vi "RTHost.vi"() -> ()   [LabVIEW 2013]
uses:
  <vilib>/Platform/TimedLoop/XDataNode/timing_clust.ctl
  <vilib>/Platform/TimedLoop/XDataNode/nitl_modes.ctl
  <vilib>/Platform/TimedLoop/XDataNode/wakeup.ctl
  <vilib>/FPGAPlugInAG/sbRIO-9632/niLvFpga_Open_sbRIO-9632.vi
  <vilib>/Utility/error.llb/Error Cluster From Error Code.vi
  <vilib>/rvi/errors/niLvFpgaAdjustHostInterfaceError.vi
  <vilib>/FPGAPlugInAG/sbRIO-9632/niLvFpga_Close_sbRIO-9632.vi
  <vilib>/rvi/interface/nirviOpenFPGA/nirviOpenFPGA.xnode
  FPGA Bitfiles/VMS15_FPGATarget_RTHost_xaXps4HcxjY.lvbitx
  <vilib>/rvi/interface/nirviReadWriteControl/nirviReadWriteControl.xnode
  <vilib>/Platform/TimedLoop/XDataNode/XDataNode.xnode
  <vilib>/rvi/interface/nirviCloseFPGA/nirviCloseFPGA.xnode
  NiFpgaLv.dll
  <vilib>/Platform/TimedLoop/XDataNode/XDNodeRunTimeDep.lvlib
panel:
  out "电池过温":bool
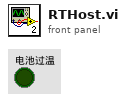
[diagram p1: front panel]
types:
  T1 = typedef "XDNodeRunTimeDep.lvlib/timing_clust.ctl" = cluster{"Expected End [f-1]":u64, "Actual End [f-1]":u64, "Finished Late? [f-1]":bool, "Expected End [i-1]":u64, "Actual End [i-1]":u64, "Finished Late? [i-1]":bool, "Expected Start [i]":u64, "Actual Start [i]":u64, "Expected Start [f]":u64, "Actual Start [f]":u64, "Source Name":string, "Structure Name":string, "Period":i64, "Deadline":i64, "Offset":i64, "Start":i64, "Priority":i32, "Timeout":i32, "Mode":T2, "Wakeup Reason":T3, "Error":errorcluster, "Source Type":string, "Secondary Source Type":string, "Global End Time":u64, "Global Start Time":u64, "Frame Duration":u64, "Iteration Duration":u64, "Assigned CPU":i32, "I/O Scan Engine Mode":u32}
  T2 = typedef "XDNodeRunTimeDep.lvlib/nitl_modes.ctl" = enum32{"No Change", "Process missed periods, maintain original phase", "Discard missed periods, maintain original phase", "Process missed periods, ignore original phase", "Discard missed periods, ignore original phase"}
  T3 = typedef "XDNodeRunTimeDep.lvlib/wakeup.ctl" = enum32{"Normal", "Aborted", "Asynchronous wakeup", "Timing source error", "Timed loop error", "Timeout"}
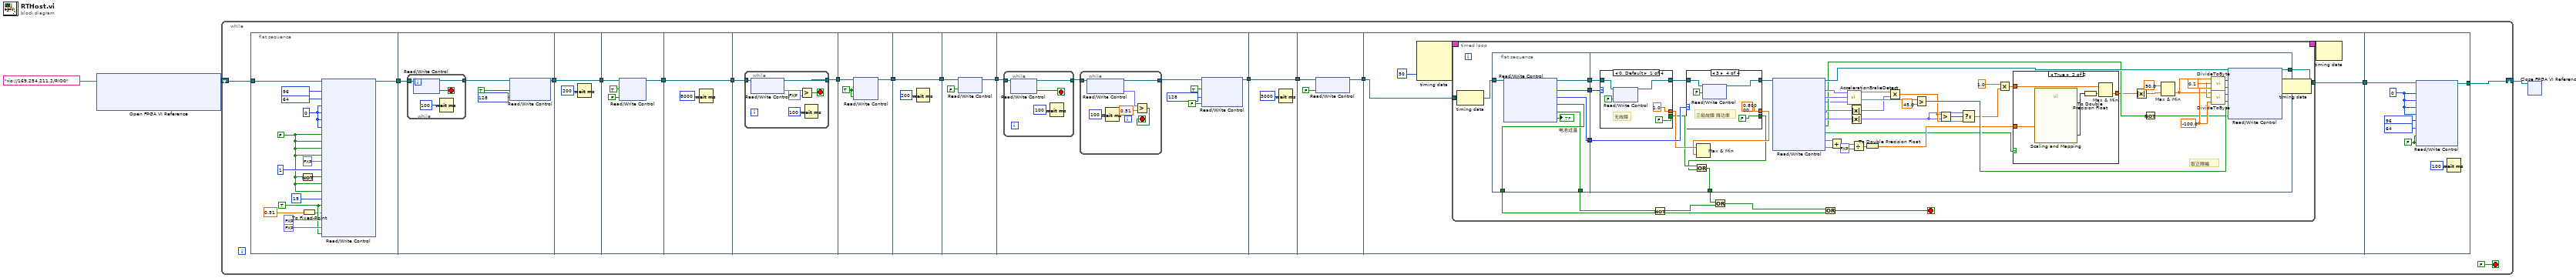
[diagram p0: block diagram]
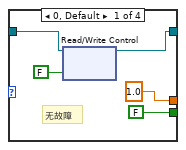
[diagram p3: hidden frame]
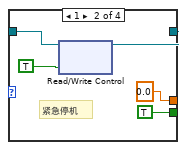
[diagram p4: hidden frame]
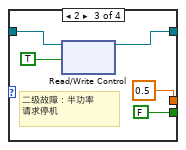
[diagram p5: hidden frame]
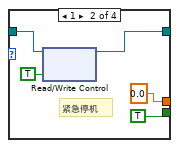
[diagram p6: hidden frame]
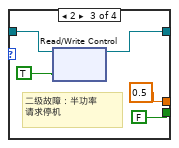
[diagram p7: hidden frame]
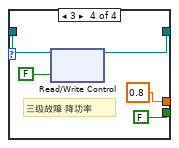
[diagram p8: hidden frame]
diagram:
  n1 = xnode "Open FPGA VI Reference"("resource name"=tag "rio://169.254.211.2/RIO0") -> ("FPGA VI Reference Out"=w1:refnum<k20>)  [unwired: 1 in, 1 out]
  n2 = while {
    shift-right: [w4] -> w2
    shift-left: w1 -> [w19]
    stop <- FALSE stop-if-true
    n3 = flat-sequence {
      tunnel: w19 -> [w31]
      tunnel: [w30] -> w18
      tunnel: w18 -> [w36]
      tunnel: [w35] -> w17
      tunnel: w17 -> [w45]
      tunnel: [w45] -> w16
      tunnel: w16 -> [w48]
      tunnel: [w47] -> w15
      tunnel: w15 -> [w51]
      tunnel: [w51] -> w10
      tunnel: [w53] -> w14
      tunnel: w10 -> [w52]
      tunnel: w14 -> [w62]
      tunnel: [w61] -> w7
      tunnel: w7 -> [w64]
      tunnel: [w64] -> w6
      tunnel: w6 -> [w67]
      tunnel: [w66] -> w5
      tunnel: w5 -> [w74]
      tunnel: [w69] -> w13
      tunnel: w13 -> [w86]
      tunnel: [w86] -> w9
      tunnel: [w88] -> w12
      tunnel: w9 -> [w89]
      tunnel: w12 -> [w92]
      tunnel: [w91] -> w11
      tunnel: w11 -> [w217]
      tunnel: [w212] -> w4
      frame #0 {
        w24 = TRUE ("AMS")
        w33 = u8 0 ("Byte 7")
        w23 = FALSE ("MotorAlarm?")
        n4 = Not(x=w23) -> (.not. x?=w22:bool)
        n5 = To Fixed-Point(number=0.51) -> (fixed-point=w21:fxp<+/-,32,16>)  [unwired: 1 in]
        n6 = xnode "Read/Write Control"("FPGA VI Reference In"=w31, "MCCmdByte"=u8 96, "BMCmdByte"=u8 64, "MC1TqSet_L"=w33, "MC1TqSet_H"=w33, "MC2TqSet_L"=w33, "MC2TqSet_H"=w33, "PREO"=w23, "AIRPO"=w23, "AIRNO"=w23, "BRAKELO"=w23, "开风扇温度值"=fxp<+,8,6> 40.0, "发送间隔(mSec)"=u8 1, "AMS"=w22, "BA"=w23, "MA"=w23, "接收窗口(mSec)"=u8 19, "Ready"=w24, "刹车标定上限"=w21, "PowerPermitted"=fxp<+/-,64,32> 60.0, "开水泵温度值"=fxp<+/-,32,16> 60.0, "ErrorMonitoring?"=w24) -> ("FPGA VI Reference Out"=w30:refnum<k20>)  [unwired: 1 in, 1 out]
      }
      frame #1 {
        n7 = while {
          tunnel: w36 -> [w43]
          tunnel: [w42] -> w37
          stop <- w40 stop-if-true
          n8 = xnode "Read/Write Control"("FPGA VI Reference In"=w43) -> ("FPGA VI Reference Out"=w42:refnum<k20>, "Start？"=w40:bool)  [unwired: 1 in, 1 out]
          n9 = Wait (ms)(milliseconds to wait=u32 100) -> ()  [unwired: 1 out]
        }
        n10 = xnode "Read/Write Control"("FPGA VI Reference In"=w37, "PREO"=TRUE, "BMCmdByte"=u8 128) -> ("FPGA VI Reference Out"=w35:refnum<k20>)  [unwired: 1 in, 1 out]
      }
      frame #2 {
        n11 = Wait (ms)(milliseconds to wait=u32 200) -> ()  [unwired: 1 out]
      }
      frame #3 {
        n12 = xnode "Read/Write Control"("FPGA VI Reference In"=w48, "AIRNO"=TRUE, "Ready"=FALSE) -> ("FPGA VI Reference Out"=w47:refnum<k20>)  [unwired: 1 in, 1 out]
      }
      frame #4 {
        n13 = Wait (ms)(milliseconds to wait=u32 8000) -> ()  [unwired: 1 out]
      }
      frame #5 {
        n14 = while {
          tunnel: [w59] -> w53
          tunnel: w52 -> [w56]
          stop <- w54 stop-if-true
          n15 = xnode "Read/Write Control"("FPGA VI Reference In"=w56) -> ("FPGA VI Reference Out"=w59:refnum<k20>, "MC1VinIs"=w57:fxp<+/-,32,16>)  [unwired: 1 in, 1 out]
          n16 = Greater?(x=w57, y=fxp<+,18,10> 480.0) -> (0:w54:bool)
          n17 = Wait (ms)(milliseconds to wait=u32 100) -> ()  [unwired: 1 out]
        }
      }
      frame #6 {
        w60 = TRUE ("AIRPO")
        n18 = xnode "Read/Write Control"("FPGA VI Reference In"=w62, "AIRPO"=w60, "Ready"=w60) -> ("FPGA VI Reference Out"=w61:refnum<k20>)  [unwired: 1 in, 1 out]
      }
      frame #7 {
        n19 = Wait (ms)(milliseconds to wait=u32 200) -> ()  [unwired: 1 out]
      }
      frame #8 {
        n20 = xnode "Read/Write Control"("FPGA VI Reference In"=w67, "PREO"=FALSE) -> ("FPGA VI Reference Out"=w66:refnum<k20>)  [unwired: 1 in, 1 out]
      }
      frame #9 {
        n21 = while {
          tunnel: w74 -> [w78]
          tunnel: [w77] -> w73
          stop <- w75 stop-if-true
          n22 = xnode "Read/Write Control"("FPGA VI Reference In"=w78) -> ("FPGA VI Reference Out"=w77:refnum<k20>, "Start？"=w75:bool)  [unwired: 1 in, 1 out]
          n23 = Wait (ms)(milliseconds to wait=u16 100) -> ()  [unwired: 1 out]
        }
        n24 = while {
          tunnel: w73 -> [w82]
          tunnel: [w81] -> w72
          stop <- w79 stop-if-true
          n25 = xnode "Read/Write Control"("FPGA VI Reference In"=w82) -> ("FPGA VI Reference Out"=w81:refnum<k20>, "SIG_BRAKE"=w80:fxp<+/-,30,9>)  [unwired: 1 in, 1 out]
          n26 = Wait (ms)(milliseconds to wait=u16 100) -> ()  [unwired: 1 out]
          n27 = Greater?(x=w80, y=0.51) -> (0:w79:bool)
        }
        n28 = xnode "Read/Write Control"("FPGA VI Reference In"=w72, "BUZZERO"=TRUE, "MCCmdByte"=u8 128 ("CAN 4"), "Ready"=FALSE) -> ("FPGA VI Reference Out"=w69:refnum<k20>)  [unwired: 1 in, 1 out]
      }
      frame #10 {
        n29 = Wait (ms)(milliseconds to wait=u32 3000) -> ()  [unwired: 1 out]
      }
      frame #11 {
        n30 = xnode "Read/Write Control"("FPGA VI Reference In"=w89, "BUZZERO"=FALSE) -> ("FPGA VI Reference Out"=w88:refnum<k20>)  [unwired: 1 in, 1 out]
      }
      frame #12 {
        n31 = node-c288(i64 50 ("Period")) -> (w94:T1)  [unwired: 3 in]
        n32 = timed-loop {
          timing: w94 -> [_]
          timing-out: [_] -> w93
          tunnel: w92 -> [w104]
          tunnel: [w105] -> w91
          stop <- w96 stop-if-true
          n33 = node-c288() -> ()  [unwired: 1 in, 1 out]
          n34 = flat-sequence {
            tunnel: w104 -> [w109]
            tunnel: [w108] -> w100
            tunnel: [w112] -> w103
            tunnel: [w111] -> w102
            tunnel: [w110] -> w101
            tunnel: [w107] -> w98
            tunnel: w103 -> [w159]
            tunnel: w102 -> [w157]
            tunnel: w101 -> [w142]
            tunnel: [w143] -> w105
            tunnel: [w119] -> w99
            frame #0 {
              n35 = xnode "Read/Write Control"("FPGA VI Reference In"=w109) -> ("FPGA VI Reference Out"=w110:refnum<k20>, "BatteryErrorRank"=w112:u8, "MotorErrorRank"=w111:u8, "Stop？"=w108:bool, "SHTD"=w107:bool, "电池过温"=→"电池过温":bool)  [unwired: 1 in, 1 out]
            }
            frame #1 {
              w150 = -100.0 ("Offset")
              w149 = 0.1 ("Resolution")
              # "取正限幅"
              n36 = case shown="0, Default" w159 {
                tunnel: [1.0 0.0 sgl 0.5 0.8] -> w156
                tunnel: [FALSE TRUE FALSE FALSE] -> w154
                tunnel: [w188 w192 w196 w201] -> w158
                tunnel: w142 -> [w187 w193 w197 w202]
                frame 0, Default {
                  # "无故障"
                  n37 = xnode "Read/Write Control"("FPGA VI Reference In"=w187, "BA"=FALSE ("Alarm")) -> ("FPGA VI Reference Out"=w188:refnum<k20>)  [unwired: 1 in, 1 out]
                }
                frame 1 {
                  # "紧急停机"
                  n38 = xnode "Read/Write Control"("FPGA VI Reference In"=w193, "BA"=TRUE) -> ("FPGA VI Reference Out"=w192:refnum<k20>)  [unwired: 1 in, 1 out]
                }
                frame 2 {
                  # "二级故障：半功率\n请求停机"
                  n39 = xnode "Read/Write Control"("FPGA VI Reference In"=w197, "BA"=TRUE ("Alarm")) -> ("FPGA VI Reference Out"=w196:refnum<k20>)  [unwired: 1 in, 1 out]
                }
                frame 3 {
                  # "三级故障 降功率"
                  n40 = xnode "Read/Write Control"("FPGA VI Reference In"=w202, "BA"=FALSE ("Alarm")) -> ("FPGA VI Reference Out"=w201:refnum<k20>)  [unwired: 1 in, 1 out]
                }
              }
              n41 = case shown="3" w157 {
                tunnel: [1.0 0.0 sgl 0.5 sgl 0.8] -> w155
                tunnel: [w169 w175 w179 w183] -> w152
                tunnel: [FALSE TRUE FALSE FALSE] -> w153
                tunnel: w158 -> [w166 w173 w176 w181]
                frame 0, Default {
                  # "无故障"
                  n42 = xnode "Read/Write Control"("FPGA VI Reference In"=w166, "MA"=FALSE ("Alarm")) -> ("FPGA VI Reference Out"=w169:refnum<k20>)  [unwired: 1 in, 1 out]
                }
                frame 1 {
                  # "紧急停机"
                  n43 = xnode "Read/Write Control"("FPGA VI Reference In"=w173, "MA"=TRUE) -> ("FPGA VI Reference Out"=w175:refnum<k20>)  [unwired: 1 in, 1 out]
                }
                frame 2 {
                  # "二级故障：半功率\n请求停机"
                  n44 = xnode "Read/Write Control"("FPGA VI Reference In"=w176, "MA"=TRUE ("Alarm")) -> ("FPGA VI Reference Out"=w179:refnum<k20>)  [unwired: 1 in, 1 out]
                }
                frame 3 {
                  # "三级故障 降功率"
                  n45 = xnode "Read/Write Control"("FPGA VI Reference In"=w181, "MA"=FALSE ("Alarm")) -> ("FPGA VI Reference Out"=w183:refnum<k20>)  [unwired: 1 in, 1 out]
                }
              }
              n46 = Or(x=w154, y=w153) -> (x .or. y?=w119:bool)
              n47 = Max & Min(x=w156, y=w155) -> ()  [unwired: 2 out]
              n48 = xnode "Read/Write Control"("FPGA VI Reference In"=w152) -> ("FPGA VI Reference Out"=w141:refnum<k20>, "SIG_ACC1"=w138:fxp<+/-,30,9>, "SIG_ACC2"=w137:fxp<+/-,30,9>, "SIG_BRAKE"=w117:fxp<+/-,30,9>, "PowerLimited"=w139:fxp<+/-,16,6>, "TorquePermitted"=w133:fxp<+/-,64,40>, "SWT3?"=w131:bool, "SWT4?"=w128:bool, "MC2SpIs"=w127:fxp<+/-,32,16>, "MC1SpIs"=w126:fxp<+/-,32,16>)  [unwired: 1 in, 1 out]
              n49 = Add(x=w127, y=w126) -> (x+y=w125:fxp<+/-,33,17>)
              n50 = call "AccelerationBrakeDetect.vi"("油门1输入"=w138, "油门2输入"=w137, "刹车输入"=w117) -> ("油门1"=w140:dbl, "刹车"=w144:dbl)  [unwired: 3 out]
              n51 = Absolute Value(x=w139) -> (abs(x)=w115:fxp<+,16,6>)
              n52 = Absolute Value(x=w133) -> (abs(x)=w116:fxp<+,64,40>)
              n53 = Divide(x=w125, y=fxp<+/-,33,17> 2.0) -> (x/y=w123:fxp<+/-,64,34>)
              n54 = To Double Precision Float(number=w123) -> (double precision float=w130:dbl)
              n55 = Multiply(x=w140, y=w115) -> (x*y=w135:dbl)
              n56 = Greater?(x=w144, y=45.0) -> (0:w136:bool)
              n57 = Greater?(x=w135, y=w116) -> (0:w134:bool)
              n58 = Select(t=w116, s=w134, f=w135) -> (s? t:f=w132:dbl)
              n59 = Multiply(x=1.0, y=w132) -> (x*y=w129:dbl)
              n60 = case shown="True" w128 {
                tunnel: w130 -> [_ w165]
                tunnel: w129 -> [w160 w161]
                tunnel: [w160 w162] -> w122
                frame False {
                }
                frame True {
                  n61 = call "Scaling and Mapping"("Signals"=w165) -> ("Scaled Signals"=w163:dynamicdata)  [unwired: 9 in, 1 out]
                  n62 = To Double Precision Float(number=w163) -> (double precision float=w164:dbl)
                  n63 = Max & Min(x=w161, y=w164) -> (min(x,y)=w162:dbl)  [unwired: 1 out]
                }
              }
              n64 = Absolute Value(x=w122) -> (abs(x)=w120:dbl)
              n65 = Not(x=w131) -> (.not. x?=w118:bool)
              n66 = Max & Min(x=90.0, y=w120) -> (min(x,y)=w114:dbl)  [unwired: 1 out]
              n67 = call "DivideToByte.vi"("Offset"=w150, "Resolution"=w149, "Value"=w114) -> ("HighByte"=w145:u8, "LowByte"=w148:u8)
              n68 = call "DivideToByte.vi"("Offset"=w150, "Resolution"=w149, "Value"=w114) -> ("HighByte"=w146:u8, "LowByte"=w147:u8)
              n69 = xnode "Read/Write Control"("FPGA VI Reference In"=w141, "MC1TqSet_L"=w148, "MC1TqSet_H"=w145, "MC2TqSet_L"=w147, "MC2TqSet_H"=w146, "BRAKELO"=w136, "ErrorMonitoring?"=w118) -> ("FPGA VI Reference Out"=w143:refnum<k20>)  [unwired: 1 in, 1 out]
            }
          }
          n70 = Not(x=w98) -> (.not. x?=w97:bool)
          n71 = Or(x=w99, y=w97) -> (x .or. y?=w95:bool)
          n72 = Or(x=w95, y=w100) -> (x .or. y?=w96:bool)
          n73 = node-c288() -> ()  [unwired: 1 in, 1 out]
        }
        n74 = node-c288(w93) -> ()  [unwired: 1 out]
      }
      frame #13 {
        w213 = FALSE ("AIRNO")
        w216 = u8 0 ("CAN 0")
        n75 = xnode "Read/Write Control"("FPGA VI Reference In"=w217, "MC1TqSet_L"=w216, "MC1TqSet_H"=w216, "MC2TqSet_L"=w216, "MC2TqSet_H"=w216, "MCCmdByte"=u8 96 ("CAN 5"), "BMCmdByte"=u8 64 ("CAN 4"), "AIRPO"=w213, "AIRNO"=w213) -> ("FPGA VI Reference Out"=w212:refnum<k20>)  [unwired: 1 in, 1 out]
        n76 = Wait (ms)(milliseconds to wait=u32 100) -> ()  [unwired: 1 out]
      }
    }
  }
  n77 = xnode "Close FPGA VI Reference"("FPGA VI Reference In"=w2) -> ()  [unwired: 1 in, 1 out]
